vi "extract From Input Packet ADC.vi"(10 "channel":i32, 11 "instance":i32) -> (3 "function return":i16)   [LabVIEW 2022 SP3, in "SADI_FW3.lvlib"]
doc: "SADI_API_Wrapper int16_t extractFromInputPacket_ADC(int instance,int channel);\nSADI_API_Wrapper uint16_t extractFromInputPacket_ADC(int instance,int channel);"
uses:
  SADI_FW3.lvlib
  SADI_FW3.dll
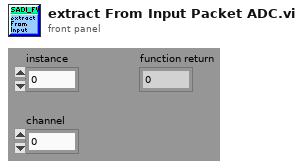
[diagram p1: front panel]
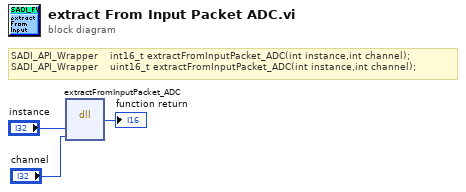
[diagram p0: block diagram]
diagram:
  # "SADI_API_Wrapper    int16_t extractFromInputPacket_ADC(int instance,int channel);\nSADI_API_Wrapper    uint16_t extractFromInputPacket_ADC(int instance,int channel);"
  n1 = dll-call lib="C:/Users/scer/OneDrive - University of Florida/eml4314c/eml4314SP23/resources/release_2_3_23/LV/LVLib/SADI_FW3.*" fn="extractFromInputPacket_ADC"("instance"="instance", "channel"="channel") -> (→"function return":i16)  [unwired: 5 in, 2 out]
